vi "Build Invert Numeric Functions.vi"   [LabVIEW 2021]
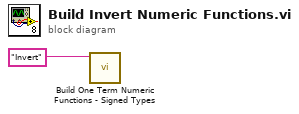
[diagram p0: block diagram]
diagram:
  n1 = call "Build One Term Numeric Functions - Signed Types.vi"("Function Name"="Invert" ("Comparison Name")) -> ()  [unwired: 11 in]
